vi "TagDB-Delete.vi"   [LabVIEW 2017, in "TagDB.lvlib"]
uses:
  TagDB.lvlib
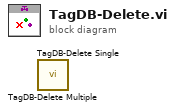
[diagram p0: block diagram]
diagram:
  n1 = call "TagDB-Delete Multiple.vi"() -> ()  [unwired: 10 in, 2 out]
  n2 = call "TagDB-Delete Single.vi"() -> ()  [unwired: 10 in, 2 out]
